vi "Enqueue.vi"(6 "Enum":enum16{"Else", "LE"}(ring), 7 "Priority (F)":bool, 8 "error in (no error)":errorcluster, 9 "Message Data":variant, 10 "Message":string, 11 "MessageQueue":refnum<queue>) -> (0 "error out":errorcluster, 3 "MessageQueue":refnum<queue>)   [LabVIEW 2018, in "SensorModule.lvlib"]
uses:
  SensorModule.lvlib
  PublicAPI/Arguments/Messages/clMessage.ctl
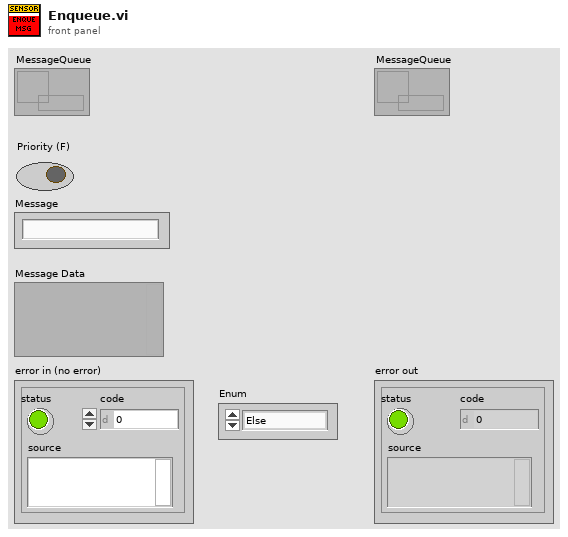
[diagram p1: front panel]
types:
  T1 = typedef "SensorModule.lvlib/clMessage.ctl" = cluster{"Message":string, "Message Data":variant}
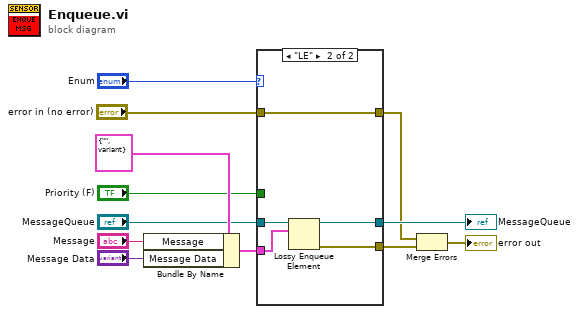
[diagram p0: block diagram]
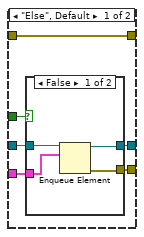
[diagram p2: hidden frame]
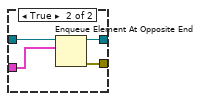
[diagram p3: hidden frame]
diagram:
  n1 = Bundle By Name(cluster=T1 {"Message"="", "Message Data"=variant} ("clMessage"), "Message"="Message", "Message Data"="Message Data") -> (w11:T1)
  n2 = case shown="\"LE\"" "Enum" {
    tunnel: w11 -> [w18 w30]
    tunnel: "MessageQueue" -> [w17 w31]
    tunnel: [w16 w28] -> w7
    tunnel: [w15 w29] -> w6
    tunnel: "Priority (F)" -> [w14 _]
    tunnel: "error in (no error)" -> [w13 w27]
    tunnel: [w13 w27] -> w1
    frame "Else", Default {
      n3 = case shown="False" w14 {
        tunnel: w18 -> [w21 w26]
        tunnel: w17 -> [w22 w25]
        tunnel: [w19 w24] -> w16
        tunnel: [w20 w23] -> w15
        frame False {
          n4 = Enqueue Element(queue=w22, element=w21) -> (queue out=w19:refnum<queue>, error out=w20:errorcluster)  [unwired: 2 in, 1 out]
        }
        frame True {
          n5 = Enqueue Element At Opposite End(queue=w25, element=w26) -> (queue out=w24:refnum<queue>, error out=w23:errorcluster)  [unwired: 2 in, 1 out]
        }
      }
    }
    frame "LE" {
      n6 = Lossy Enqueue Element(queue=w31, element=w30) -> (queue out=w28:refnum<queue>, error out=w29:errorcluster)  [unwired: 1 in, 2 out]
    }
  }
  "MessageQueue" <- w7
  n7 = Merge Errors(w1, w6) -> (→"error out":errorcluster)
